vi "pcfs_check_stop_queue.vi"(8 "error in (no error)":errorcluster, 11 "scan_panel in":refnum<class "pcfs.lvclass">) -> (0 "error out":errorcluster, 2 "stop?":bool, 3 "scan_panel out":refnum<class "pcfs.lvclass">)   [LabVIEW 2015, in "pcfs.lvclass"]
uses:
  pcfs.lvclass
  pcfs.lvclass/pcfs.ctl
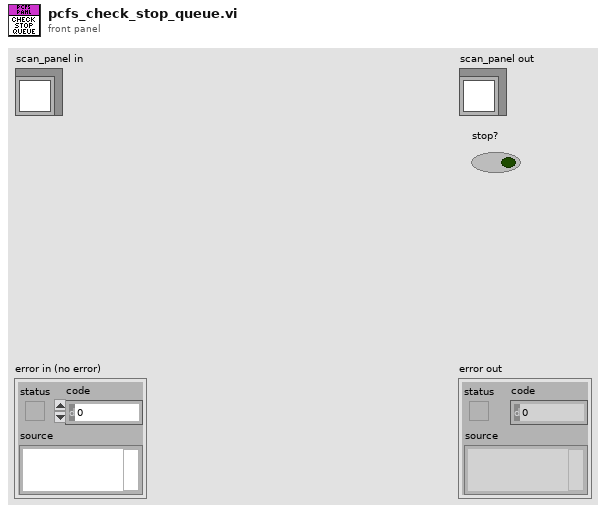
[diagram p1: front panel]
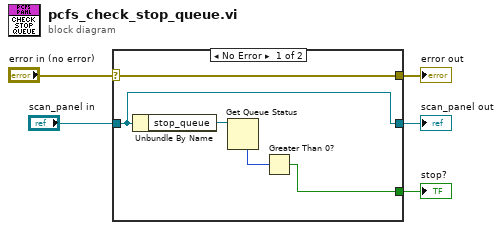
[diagram p0: block diagram]
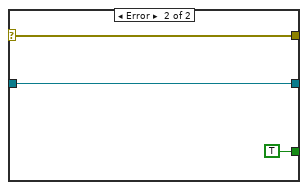
[diagram p2: hidden frame]
diagram:
  n1 = case shown="No Error" "error in (no error)" {
    selector: "error in (no error)" -> [w10 w13]
    tunnel: [w10 w13] -> w4
    tunnel: [w9 w12] -> w2
    tunnel: "scan_panel in" -> [w9 w12]
    tunnel: [w6 TRUE] -> w1
    frame No Error {
      n2 = Unbundle By Name(w9) -> ("stop_queue"=w8:refnum<queue>)
      n3 = Get Queue Status(queue=w8) -> (# elements in queue=w7:i32)  [unwired: 2 in, 7 out]
      n4 = Greater Than 0?(x=w7) -> (x > 0?=w6:bool)
    }
    frame Error {
    }
  }
  "error out" <- w4
  "scan_panel out" <- w2
  "stop?" <- w1
